vi "ConvertTextBasedCodeToLabVIEW_CreateCommonItems.vi"(8 "error in (no error)":errorcluster, 11 "MissingItems":T1[](array[typedef])) -> (0 "error out":errorcluster, 1 "EnumsOusideClass":T13[](array[typedef]), 2 "StructsOusideClass":T14[](array[typedef]), 3 "Classes":T3[](array[typedef]), 4 "NothingAdded":bool)   [LabVIEW 2020]
uses:
  CommonVIs/CommonVIs_EnumType.ctl
  String/GDSString_AccessScopeModifierType.ctl
  String/GDSString_ModifierType.ctl
  CommonVIs/CommonVIs_StructType.ctl
  CommonVIs/CommonVIs_AttributeType.ctl
  CommonVIs/CommonVIs_AttributeDataType.ctl
  String/GDSString_ClassDescriptionType.ctl
  String/GDSString_MethodDescriptionType.ctl
  CommonVIs/CommonVIs_PropertyType.ctl
  String/GDSString_ClassParentType.ctl
  String/GDSString_ClassType.ctl
  String/GDSString_ClassOwnerType.ctl
  ConvertTextBasedCodeToLabVIEW_MissingType.ctl
  ConvertTextBasedCodeToLabVIEW_MissingTypeIconType.ctl
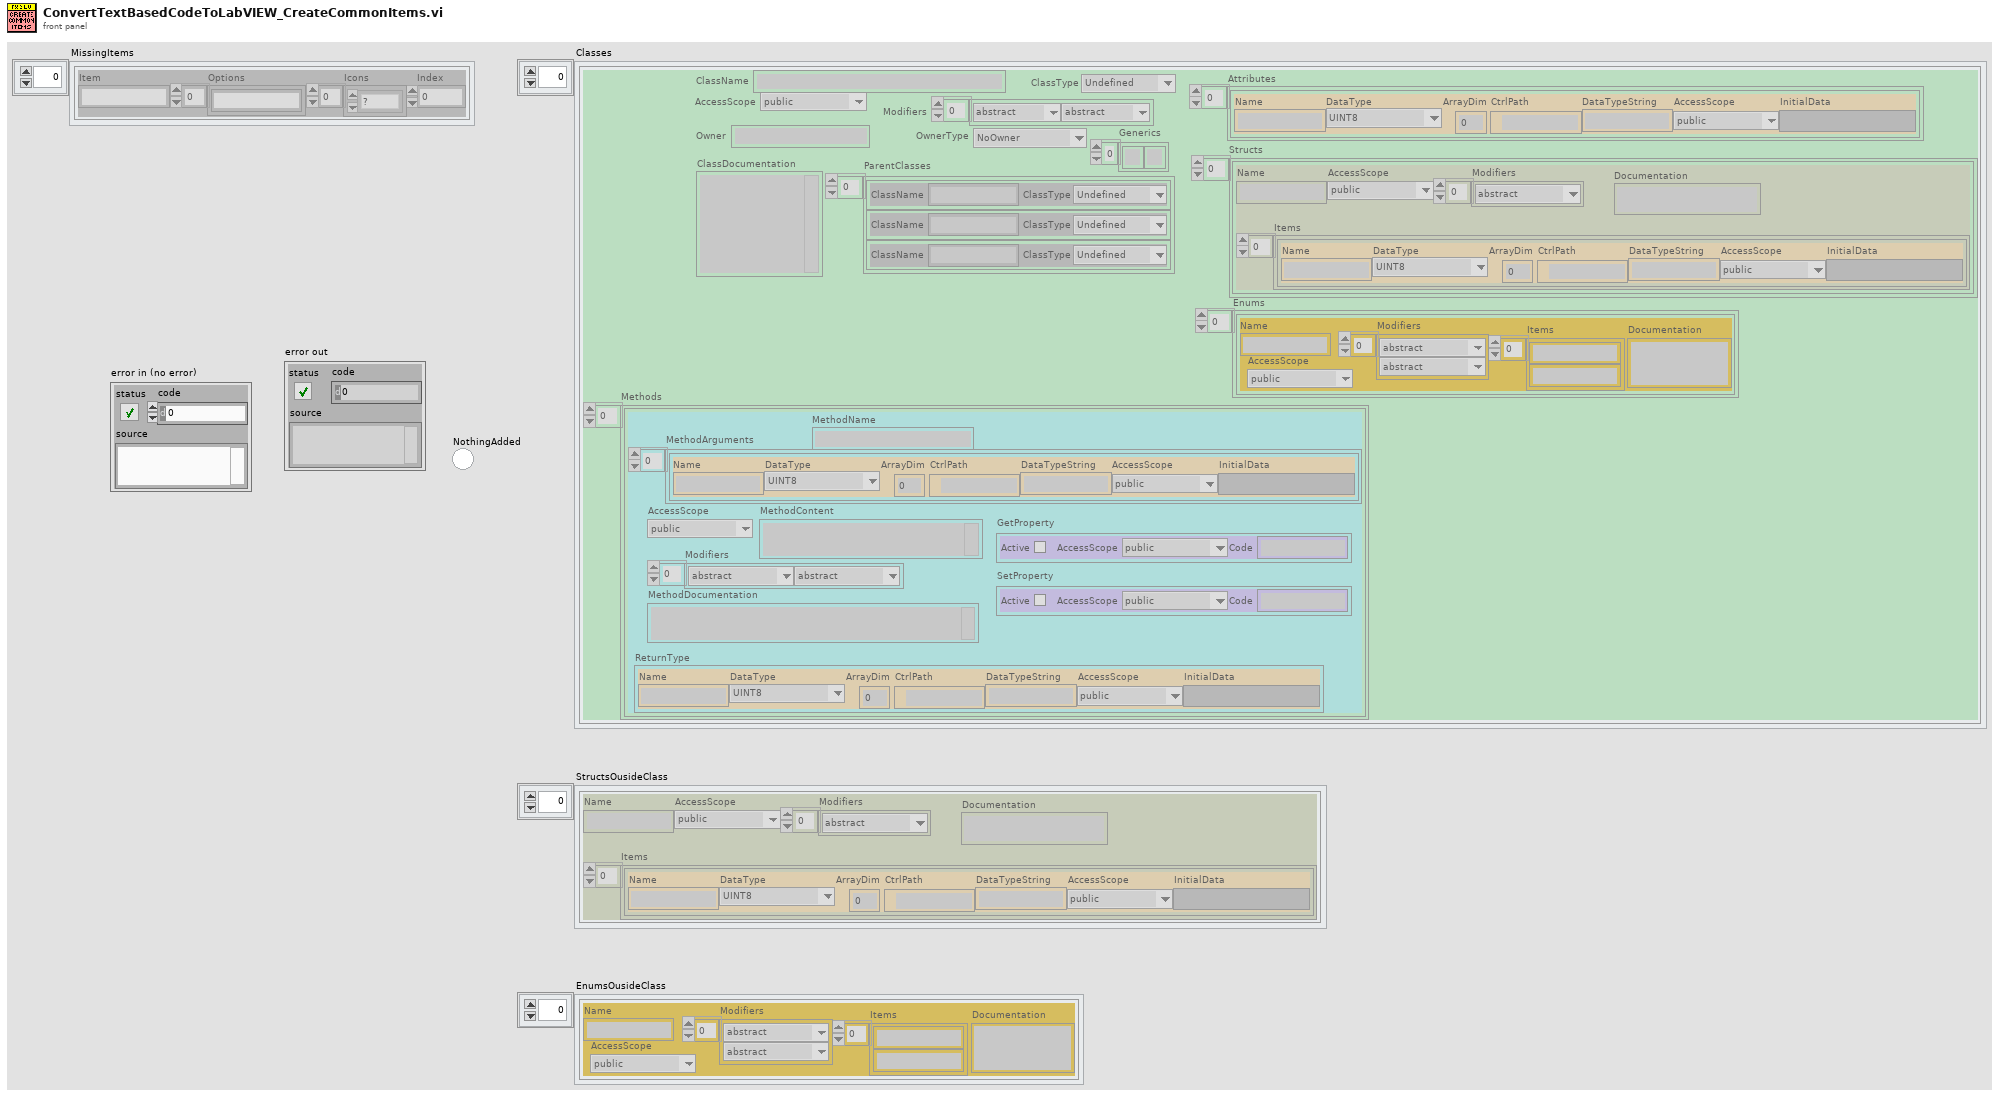
[diagram p1: front panel]
types:
  T1 = typedef "ConvertTextBasedCodeToLabVIEW_MissingType.ctl" = cluster{"Item":string, "Options":string[], "Icons":T2[], "Index":i32}
  T2 = typedef "ConvertTextBasedCodeToLabVIEW_MissingTypeIconType.ctl" = enum16{"?", "Add", "Delete", "Implement", "Inherit"}
  T3 = typedef "GDSString_ClassDescriptionType.ctl" = cluster{"ClassName":string, "AccessScope":T4, "Modifiers":T5[], "ClassDocumentation":string, "Methods":T6[], "ParentClasses":T10[], "ClassType":T11, "Owner":string, "OwnerType":T12, "Generics":string[], "Attributes":T7[], "Enums":T13[], "Structs":T14[]}
  T4 = typedef "GDSString_AccessScopeModifierType.ctl" = enum16{"public", "private", "protected", "internal"}
  T5 = typedef "GDSString_ModifierType.ctl" = enum16{"abstract", "static", "final", "synchronized", "strictfp", "async", "const", "event", "extern", "new", "native ", "override", "partial", "readonly", "sealed", "unsafe", "virtual", "volatile"}
  T6 = typedef "GDSString_MethodDescriptionType.ctl" = cluster{"ReturnType":T7, "MethodName":string, "AccessScope":T4, "Modifiers":T5[], "MethodDocumentation":string, "MethodContent":string, "MethodArguments":T7[], "GetProperty":T9, "SetProperty":T9}
  T7 = typedef "CommonVIs_AttributeType.ctl" = cluster{"Name":string, "DataType":T8, "ArrayDim":i32, "CtrlPath":path, "DataTypeString":string, "AccessScope":T4, "InitialData":variant}
  T8 = typedef "CommonVIs_AttributeDataType.ctl" = enum16{"UINT8", "INT8", "UINT16", "INT16", "UINT32", "INT32", "UINT64", "INT64", "SGL", "DBL", "EXT", "CSG", "CDB", "CXT", "TimeStamp", "STRING", "PATH", "BOOL", "ENUM", "RefNum", "VIRefNum", "LabVIEW Class", "Cluster", "Variant", "TypeDef", "Waveform", "LabVIEW Object", "Other", "void", "Set", "Map"}
  T9 = typedef "CommonVIs_PropertyType.ctl" = cluster{"Active":bool, "AccessScope":T4, "Code":string}
  T10 = typedef "GDSString_ClassParentType.ctl" = cluster{"ClassName":string, "ClassType":T11}
  T11 = typedef "GDSString_ClassType.ctl" = enum16{"Undefined", "Class", "Interface"}
  T12 = typedef "GDSString_ClassOwnerType.ctl" = enum16{"NoOwner", "Class", "Package/NameSpace"}
  T13 = typedef "CommonVIs_EnumType.ctl" = cluster{"Name":string, "AccessScope":T4, "Modifiers":T5[], "Items":string[], "Documentation":string}
  T14 = typedef "CommonVIs_StructType.ctl" = cluster{"Name":string, "AccessScope":T4, "Modifiers":T5[], "Items":T7[], "Documentation":string}
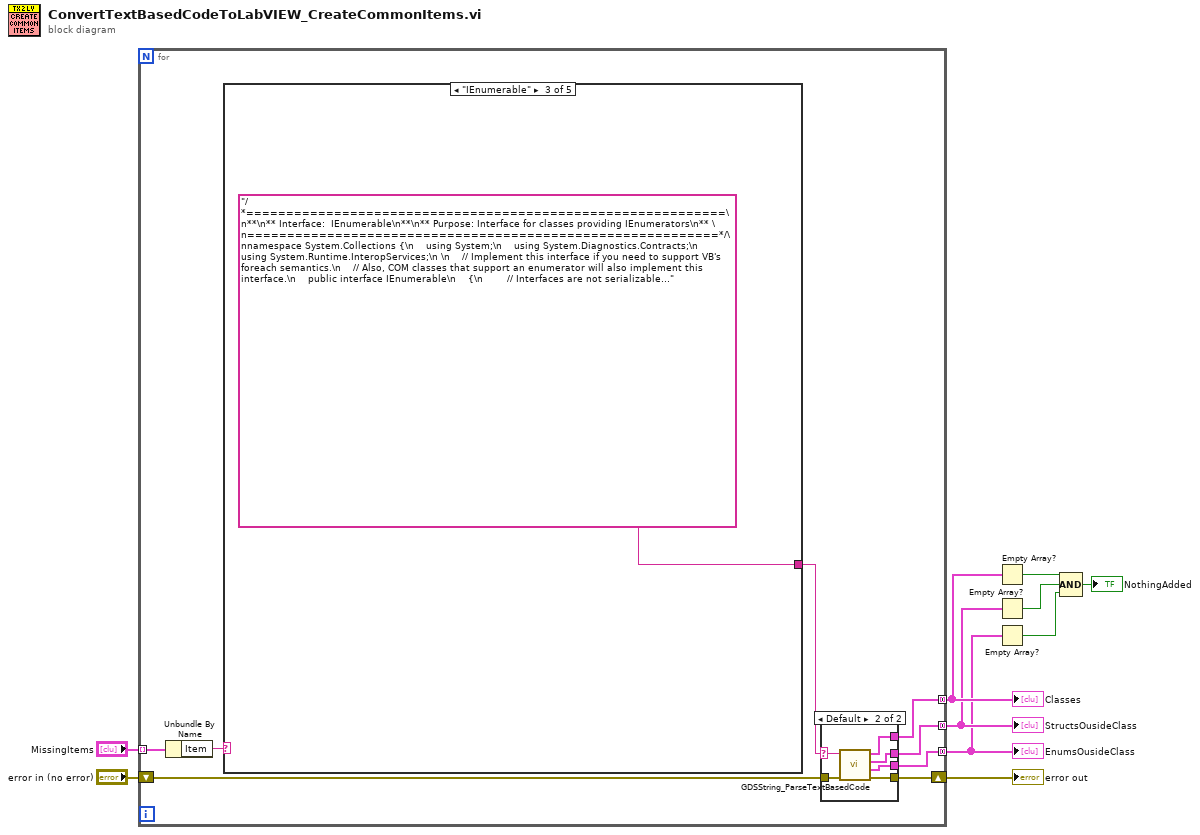
[diagram p0: block diagram]
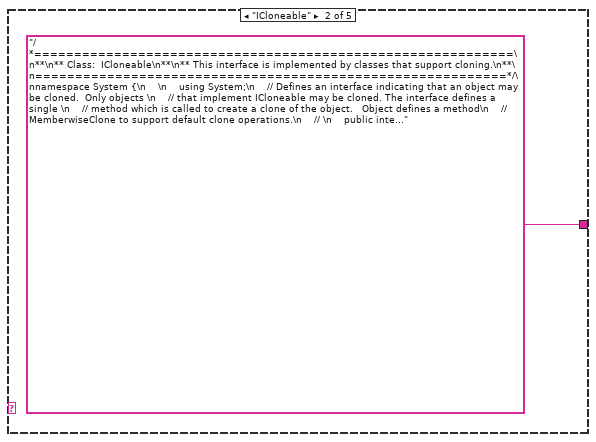
[diagram p4: hidden frame]
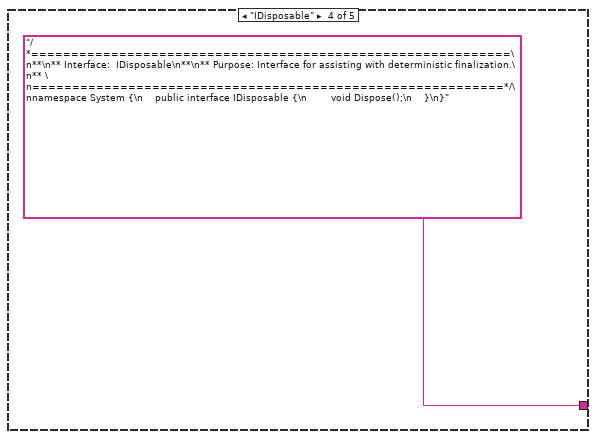
[diagram p5: hidden frame]
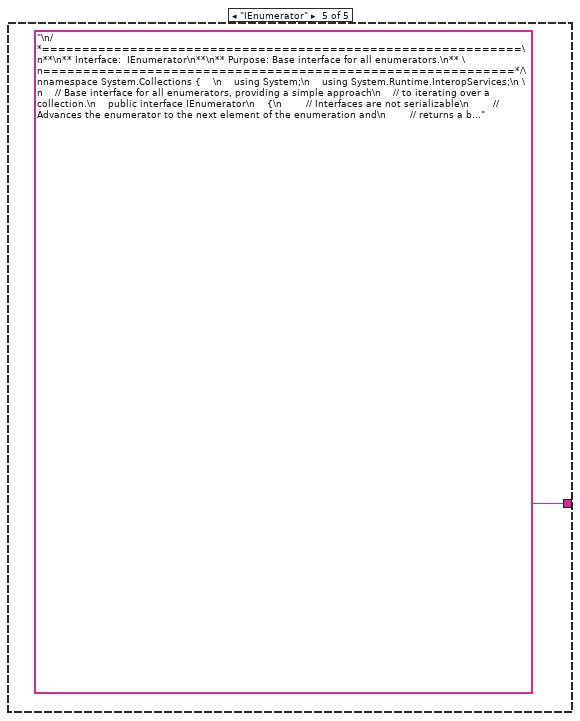
[diagram p6: hidden frame]
diagram:
  n1 = for {
    tunnel: [w18] -> w5 mode=concatenating
    tunnel: [w17] -> w6 mode=concatenating
    tunnel: [w16] -> w7 mode=concatenating
    shift-right: [w14] -> w9
    shift-left: "error in (no error)" -> [w15]
    tunnel: "MissingItems" -> [w13] mode=indexing
    n2 = Unbundle By Name(w13) -> ("Item"=w12:string)
    n3 = case shown="\"IEnumerable\"" w12 {
      tunnel: [_ "/*============================================================\n**\n** Class:  ICloneable\n**\n** This interface is implemented by classes that support cloning.\n**\n===========================================================*/\nnamespace System {\n    \n    using System;\n    // Defines an interface indicating that an object may be cloned.  Only objects \n    // that implement ICloneable may be cloned. The interface defines a single \n    // method which is called to create a clone of the object.   Object defines a method\n    // MemberwiseClone to support default clone operations.\n    // \n    public interface ICloneable\n    {\n        // Interface does not need to be marked with the serializable attribute\n        // Make a new object which is a copy of the object instanced.  This object may be either\n        // deep copy or a shallow copy depending on the implementation of clone.  The default\n        // Object support for clone does a shallow copy.\n        // \n        Object Clone();\n    }\n}" "/*============================================================\n**\n** Interface:  IEnumerable\n**\n** Purpose: Interface for classes providing IEnumerators\n** \n===========================================================*/\nnamespace System.Collections {\n    using System;\n    using System.Diagnostics.Contracts;\n    using System.Runtime.InteropServices;\n \n    // Implement this interface if you need to support VB's foreach semantics.\n    // Also, COM classes that support an enumerator will also implement this interface.\n    public interface IEnumerable\n    {\n        // Interfaces are not serializable\n        // Returns an IEnumerator for this enumerable Object.  The enumerator provides\n        // a simple way to access all the contents of a collection.\n        IEnumerator GetEnumerator();\n    }\n }" "/*============================================================\n**\n** Interface:  IDisposable\n**\n** Purpose: Interface for assisting with deterministic finalization.\n** \n===========================================================*/\nnamespace System {\n    public interface IDisposable {\n        void Dispose();\n    }\n}" "\n/*============================================================\n**\n** Interface:  IEnumerator\n**\n** Purpose: Base interface for all enumerators.\n** \n===========================================================*/\nnamespace System.Collections {    \n    using System;\n    using System.Runtime.InteropServices;\n \n    // Base interface for all enumerators, providing a simple approach\n    // to iterating over a collection.\n    public interface IEnumerator\n    {\n        // Interfaces are not serializable\n        // Advances the enumerator to the next element of the enumeration and\n        // returns a boolean indicating whether an element is available. Upon\n        // creation, an enumerator is conceptually positioned before the first\n        // element of the enumeration, and the first call to MoveNext \n        // brings the first element of the enumeration into view.\n        // \n        bool MoveNext();\n    \n        // Returns the current element of the enumeration. The returned value is\n        // undefined before the first call to MoveNext and following a\n        // call to MoveNext that returned false. Multiple calls to\n        // GetCurrent with no intervening calls to MoveNext \n        // will return the same object.\n        // \n        Object Current {\n            get; \n        }\n    \n        // Resets the enumerator to the beginning of the enumeration, starting over.\n        // The preferred behavior for Reset is to return the exact same enumeration.\n        // This means if you modify the underlying collection then call Reset, your\n        // IEnumerator will be invalid, just as it would have been if you had called\n        // MoveNext or Current.\n        //\n        void Reset();\n    }\n}"] -> w11
      frame Default {
      }
      frame "ICloneable" {
      }
      frame "IEnumerable" {
      }
      frame "IDisposable" {
      }
      frame "IEnumerator" {
      }
    }
    n4 = case shown="Default" w11 {
      selector: w11 -> [_ w20]
      tunnel: [_ w25] -> w18
      tunnel: [_ w24] -> w17
      tunnel: [_ w23] -> w16
      tunnel: w15 -> [w19 w22]
      tunnel: [w19 w21] -> w14
      frame "" {
      }
      frame Default {
        n5 = call "GDSString_ParseTextBasedCode.vi"("error in (no error)"=w22, "TextIn"=w20) -> ("error out"=w21:errorcluster, "EnumsOusideClass"=w25:T13[], "StructsOusideClass"=w24:T14[], "Classes"=w23:T3[])  [unwired: 6 in]
      }
    }
  }
  "EnumsOusideClass" <- w5
  "StructsOusideClass" <- w6
  "Classes" <- w7
  "error out" <- w9
  n6 = Empty Array?(array=w7) -> (empty?=w4:bool)
  n7 = Empty Array?(array=w6) -> (empty?=w3:bool)
  n8 = Empty Array?(array=w5) -> (empty?=w2:bool)
  n9 = Compound Arithmetic op=AND(w4, w3, w2) -> (→"NothingAdded":bool)
